vi "Test 1.vi"() -> ()   [LabVIEW 2016]
uses:
  <vilib>/Rock Robotics/WPI/SafetyOutput/WPI_SafetyOutputConfigMenu.ctl
panel:
  in  "Drive Effort":dbl=1000.0
  in  "Duration":u32=3500
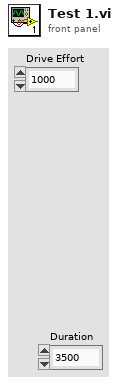
[diagram p1: front panel]
types:
  T1 = typedef "WPI_SafetyOutputConfigMenu.ctl" = enum16{"Enable", "Disable"}
  T2 = typedef "WPI_MotorControlDeviceRef.ctl" = cluster{"DeviceStatus":errorcluster, "Type":T3, "PWM":cluster{"PWM Channel":T4, "DeadBand":T5}, "CAN":cluster{"Device Number":u8, "SetOutput VI Ref":variant, "GetOutput VI Ref":variant, "Enable VI Ref":variant, "Disable VI Ref":variant, "Data":variant}, "Invert":bool}
  T3 = typedef "WPI_MotorControlType.ctl" = enum16{"PWM", "CAN"}
  T4 = typedef "FPGA_DIOPWMChannel.ctl" = enum8{"PWM 0", "PWM 1", "PWM 2", "PWM 3", "PWM 4", "PWM 5", "PWM 6", "PWM 7", "PWM 8", "PWM 9", "PWM MXP 0", "PWM MXP 1", "PWM MXP 2", "PWM MXP 3", "PWM MXP 4", "PWM MXP 5", "PWM MXP 6", "PWM MXP 7", "PWM MXP 8", "PWM MXP 9", "Invalid"}
  T5 = typedef "WPI_PWMDeadband.ctl" = cluster{"Name":string, "maxPositivePwm":i32, "minPositivePwm":i32, "centerPwm":i32, "maxNegativePwm":i32, "minNegativePwm":i32, "angularRange":u16}
  T6 = typedef "WPI_CANTalonSRX_GlobalStatus.ctl" = cluster{"Applied Throttle":dbl, "Module Enabled":bool, "CAN Error":errorcluster, "Closed Loop Error":dbl, "Forward Limit Switch Closed":bool, "Reverse Limit Switch Closed":bool, "Sensor Position":dbl, "Sensor Velocity":dbl, "Current":dbl, "Sticky Fault - Over Temp":bool, "Sticky Fault - Under Voltage":bool, "Sticky Fault - Forward Limit":bool, "Sticky Fault - Reverse Limit":bool, "Sticky Fault - Forward Soft Limit":bool, "Sticky Fault - Reverse Soft Limit":bool, "Brake is Enabled":bool, "Encoder Position":dbl, "Encoder Velocity":dbl, "Encoder Index Count":dbl, "Encoder A Pin State":bool, "Encoder B Pin State":bool, "Encoder Index Pin State":bool, "Analog In":dbl, "Analog In Velocity":dbl, "Temperature (C)":dbl, "Battery Voltage":dbl, "Control 5 Is Supported":bool, "Current Profile Slot Select":dbl, "Pos Div 8":bool, "Vel Div 4":bool, "Pulse Width Position":i32, "Pulse Width Velocity":i32, "Pulse Width Rise To Rise (us)":i32, "Pulse Width Rise To Fall (us)":i32, "Mot Prof Active Is Under Run":bool, "Mot Prof Active Has Under Run":bool, "Mot Prof Active Is Last":bool, "Mot Prof Active Velocity Only":bool, "Mot Prof Active Is Valid":bool, "Mot Prof Buffer Is Full":bool, "Mot Prof Active Profile Slot Select":i32, "Mot Prof NextID":i32, "Mot Prof Count":i32, "Mot Prof Active Velocity":dbl, "Mot Prof Active Position":dbl, "Mot Prof Output Enable":i32}
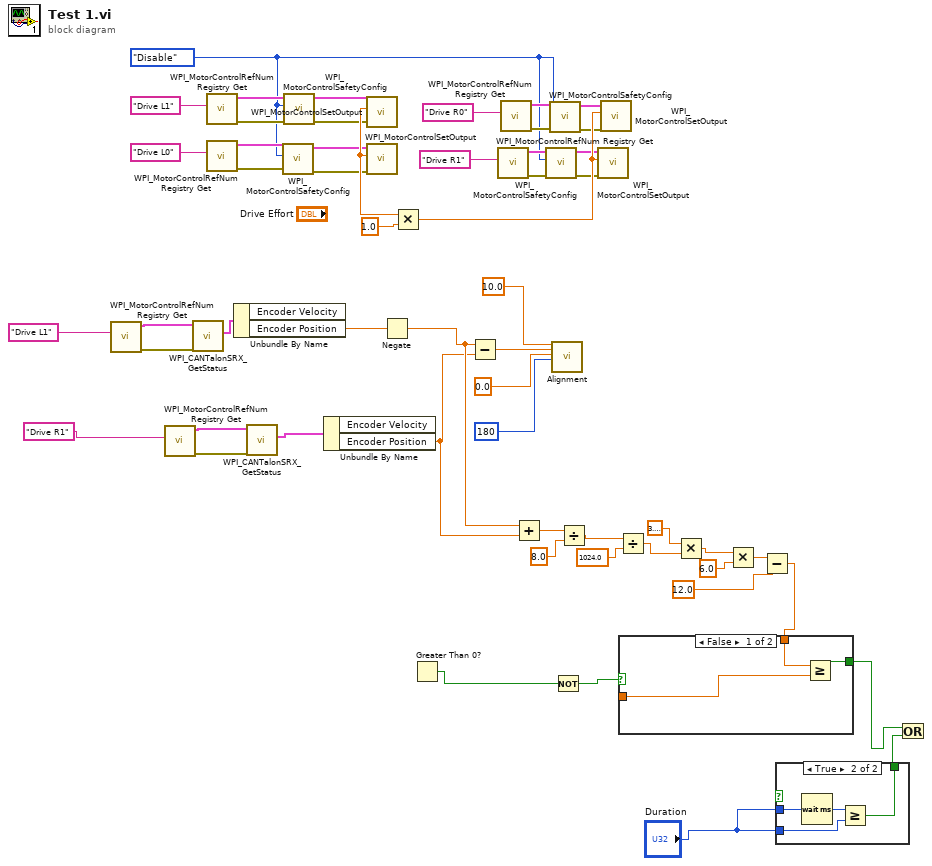
[diagram p0: block diagram]
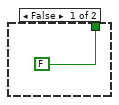
[diagram p2: hidden frame]
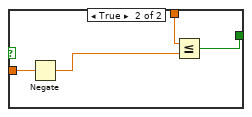
[diagram p3: hidden frame]
diagram:
  w1 = WPI_SafetyOutputConfigMenu."Disable" ("mode")
  n1 = call <vilib>:"WPI_MotorControlRefNum Registry Get.vi"("refnum name"="Drive L1") -> ("error out"=w51:errorcluster, "MotorControlDevRef"=w56:T2)  [unwired: 9 in]
  n2 = call <vilib>:"WPI_MotorControlRefNum Registry Get.vi"("refnum name"="Drive R1") -> ("error out"=w54:errorcluster, "MotorControlDevRef"=w55:T2)  [unwired: 9 in]
  n3 = call <vilib>:"WPI_CANTalonSRX_GetStatus.vi"("error in (no error)"=w51, "CAN Talon SRX Ref"=w56) -> ("Talon SRX Status"=w53:T6)  [unwired: 7 in, 2 out]
  n4 = call <vilib>:"WPI_MotorControlRefNum Registry Get.vi"("refnum name"="Drive L1") -> ("error out"=w16:errorcluster, "MotorControlDevRef"=w17:T2)  [unwired: 9 in]
  n5 = call <vilib>:"WPI_MotorControlRefNum Registry Get.vi"("refnum name"="Drive L0") -> ("error out"=w12:errorcluster, "MotorControlDevRef"=w13:T2)  [unwired: 9 in]
  n6 = Unbundle By Name(w53) -> ("Encoder Position"=w47:dbl)  [unwired: 1 out]
  n7 = call <vilib>:"WPI_CANTalonSRX_GetStatus.vi"("error in (no error)"=w54, "CAN Talon SRX Ref"=w55) -> ("Talon SRX Status"=w52:T6)  [unwired: 7 in, 2 out]
  n8 = call <vilib>:"WPI_MotorControlSafetyConfig.vi"("error in (no error)"=w12, "mode"=w1, "MotorControlDevRef"=w13) -> ("error out"=w10:errorcluster, "MotorControlDevRef"=w11:T2)  [unwired: 7 in]
  n9 = call <vilib>:"WPI_MotorControlSafetyConfig.vi"("error in (no error)"=w16, "mode"=w1, "MotorControlDevRef"=w17) -> ("error out"=w14:errorcluster, "MotorControlDevRef"=w15:T2)  [unwired: 7 in]
  n10 = Unbundle By Name(w52) -> ("Encoder Position"=w25:dbl)  [unwired: 1 out]
  n11 = call <vilib>:"WPI_MotorControlSetOutput.vi"("error in (no error)"=w14, "MotorControlDevRef"=w15) -> ("Output"=w18:dbl)  [unwired: 6 in, 3 out]
  n12 = call <vilib>:"WPI_MotorControlSetOutput.vi"("error in (no error)"=w10, "Output"=w18, "MotorControlDevRef"=w11) -> ()  [unwired: 6 in, 3 out]
  n13 = Negate(x=w47) -> (-x=w26:dbl)
  n14 = Multiply(x=w18, y=1.0) -> (x*y=w19:dbl)
  n15 = Greater Than 0?() -> (x > 0?=w32:bool)  [unwired: 1 in]
  n16 = Subtract(x=w26, y=w25) -> (x-y=w46:dbl)
  n17 = call <vilib>:"WPI_MotorControlRefNum Registry Get.vi"("refnum name"="Drive R1") -> ("error out"=w4:errorcluster, "MotorControlDevRef"=w5:T2)  [unwired: 9 in]
  n18 = call <vilib>:"WPI_MotorControlRefNum Registry Get.vi"("refnum name"="Drive R0") -> ("error out"=w8:errorcluster, "MotorControlDevRef"=w9:T2)  [unwired: 9 in]
  n19 = Add(x=w26, y=w25) -> (x+y=w43:dbl)
  n20 = call <vilib>:"WPI_MotorControlSafetyConfig.vi"("error in (no error)"=w4, "mode"=w1, "MotorControlDevRef"=w5) -> ("error out"=w3:errorcluster, "MotorControlDevRef"=w2:T2)  [unwired: 7 in]
  n21 = call <vilib>:"WPI_MotorControlSafetyConfig.vi"("error in (no error)"=w8, "mode"=w1, "MotorControlDevRef"=w9) -> ("error out"=w7:errorcluster, "MotorControlDevRef"=w6:T2)  [unwired: 7 in]
  n22 = call "Alignment.vi"("Range"=10.0, "Camera Feedback"=w46, "Target"=0.0, "POV"=180) -> ()  [unwired: 13 in, 3 out]
  n23 = Not(x=w32) -> (.not. x?=w27:bool)
  n24 = Divide(x=w43, y=8.0) -> (x/y=w41:dbl)
  n25 = call <vilib>:"WPI_MotorControlSetOutput.vi"("error in (no error)"=w3, "Output"=w19, "MotorControlDevRef"=w2) -> ()  [unwired: 6 in, 3 out]
  n26 = call <vilib>:"WPI_MotorControlSetOutput.vi"("error in (no error)"=w7, "Output"=w19, "MotorControlDevRef"=w6) -> ()  [unwired: 6 in, 3 out]
  n27 = Divide(x=w41, y=1024.0) -> (x/y=w39:dbl)
  n28 = Multiply(x=3.141592653589793, y=w39) -> (x*y=w37:dbl)
  n29 = Multiply(x=w37, y=6.0) -> (x*y=w35:dbl)
  n30 = Subtract(x=w35, y=12.0) -> (x-y=w33:dbl)
  n31 = case shown="False" w27 {
    tunnel: [w57 w63] -> w31
    tunnel: _ -> [w58 w61]
    tunnel: w33 -> [w59 w60]
    frame False {
      n32 = Greater Or Equal?(x=w59, y=w58) -> (x >= y?=w57:bool)
    }
    frame True {
      n33 = Negate(x=w61) -> (-x=w62:dbl)
      n34 = Less Or Equal?(x=w60, y=w62) -> (x <= y?=w63:bool)
    }
  }
  n35 = case shown="True" {
    selector: _ -> [_ _]
    tunnel: "Duration" -> [_ w67]
    tunnel: [FALSE w66] -> w30
    tunnel: "Duration" -> [_ w65]
    frame False {
    }
    frame True {
      n36 = Wait (ms)(milliseconds to wait=w65) -> (millisecond timer value=w68:u32)
      n37 = Greater Or Equal?(x=w68, y=w67) -> (x >= y?=w66:bool)
    }
  }
  n38 = Or(x=w31, y=w30) -> (x .or. y?=w29:bool)
